vi "Untitled 5 (SubVI).vi"(8 "error in (no error)":errorcluster, 10 "Boolean":bool, 11 "VI in":refnum<vi>) -> (0 "error out":errorcluster)   [LabVIEW 2015]
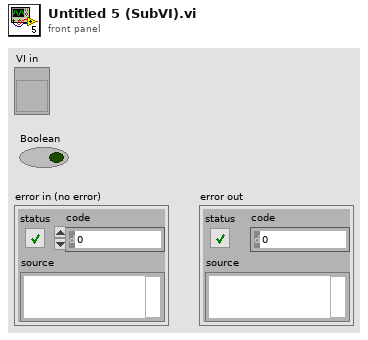
[diagram p1: front panel]
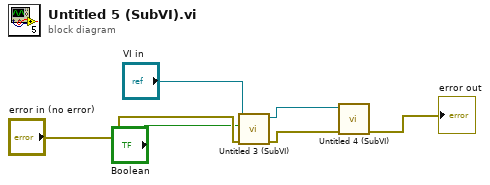
[diagram p0: block diagram]
diagram:
  n1 = call "Untitled 3 (SubVI).vi"("error in (no error)"="error in (no error)", "Boolean"="Boolean", "VI in"="VI in") -> ("error out"=w3:errorcluster, "VI out"=w2:refnum<vi>)  [unwired: 7 in]
  n2 = call "Untitled 4 (SubVI).vi"("error in (no error)"=w3, "VI in"=w2) -> ("error out"=→"error out":errorcluster)  [unwired: 9 in]
